vi "Database Transaction.vi"() -> ()   [LabVIEW 2013]
doc: "This VI demonstates the use of transactions on a table named transaxn in the LabVIEW.mdb database. \n\nA transaction is begun and then a table is created in the database. The user is then prompted to decide whether or not to commit the transaction and \"write\" the changes to the database."
uses:
  Auxilliary.llb/DB Tools Column Info.ctl
  Auxilliary.llb/DB Tools DataTypes.ctl
  Auxilliary.llb/DB Tools Transaction.ctl
  Connection.llb/DB Tools Open Connec (Path).vi
  Connection.llb/Conn Transaction.vi
  NI_Database_API_64.lvlib
panel:
  in  "column information":T1[](array[typedef])=[{"column name"="test", "data type"=enum."String", "size"=30, "allow null?"=FALSE}]
  in  "table":string="transaxn"
  # "INSTRUCTIONS:\n\nRun the VI.  A database connection is established and a table is created. A dialog box is then displayed asking if you want to commit or rollback the transaction."
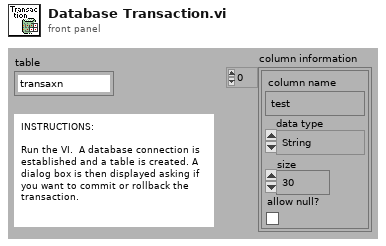
[diagram p1: front panel]
types:
  T1 = typedef "NI_Database_API_64.lvlib/DB Tools Column Info.ctl" = cluster{"column name":string, "data type":T2, "size":i32, "allow null?":bool}
  T2 = typedef "NI_Database_API_64.lvlib/DB Tools DataTypes.ctl" = enum16{"String", "Long (I32)", "Single (SGL)", "Double (DBL)", "Date/Time", "Binary"}
  T3 = typedef "NI_Database_API_64.lvlib/DB Tools Transaction.ctl" = enum16{"begin", "commit", "rollback"}
  T4 = typedef "NI_Database_API_64.lvlib/Conn ObjectReference.ctl" = refnum<k1>
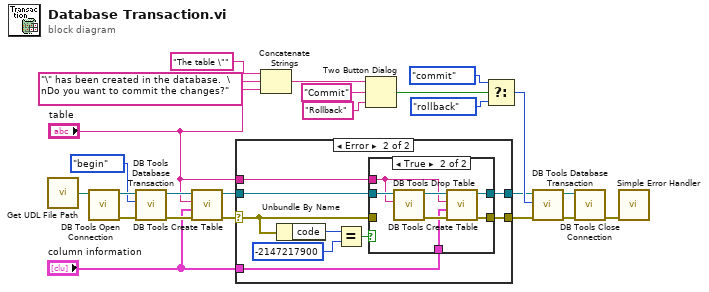
[diagram p0: block diagram]
diagram:
  n1 = call "Get UDL File Path.vi"() -> ("UDL file path"=w9:path)  [unwired: 1 in]
  n2 = call-poly "DB Tools Open Connection.vi"("connection information"=w9) -> ("error out"=w24:errorcluster, "connection reference"=w23:T4)  [unwired: 7 in]
  n3 = call-poly "DB Tools Database Transaction.vi"("error in (no error)"=w24, "operation (begin)"=DB_Tools_Transaction."begin", "connection reference"=w23) -> ("error out"=w21:errorcluster, "connection reference out"=w20:T4)  [unwired: 3 in]
  n4 = call "DB Tools Create Table.vi"("error in (no error)"=w21, "column information"="column information", "table"="table", "connection reference"=w20) -> ("error out"=w6:errorcluster, "connection reference out"=w5:T4)  [unwired: 4 in]
  n5 = case shown="Error" w6 {
    selector: w6 -> [w25 w28]
    tunnel: w5 -> [w26 w33]
    tunnel: [w26 w32] -> w4
    tunnel: [w25 w31] -> w3
    tunnel: "table" -> [_ w30]
    tunnel: "column information" -> [_ w27]
    frame No Error {
    }
    frame Error {
      n6 = Unbundle By Name(w28) -> ("code"=w35:i32)
      n7 = Equal?(x=w35, y=-2147217900) -> (x = y?=w29:bool)
      n8 = case shown="True" w29 {
        tunnel: w33 -> [w37 w44]
        tunnel: [w37 w39] -> w32
        tunnel: [w36 w38] -> w31
        tunnel: w30 -> [_ w41]
        tunnel: w28 -> [w36 _]
        tunnel: w27 -> [_ w40]
        frame False {
        }
        frame True {
          n9 = call "DB Tools Drop Table.vi"("table"=w41, "connection reference"=w44) -> ("error out"=w43:errorcluster, "connection reference out"=w42:T4)  [unwired: 6 in]
          n10 = call "DB Tools Create Table.vi"("error in (no error)"=w43, "column information"=w40, "table"=w41, "connection reference"=w42) -> ("error out"=w38:errorcluster, "connection reference out"=w39:T4)  [unwired: 4 in]
        }
      }
    }
  }
  n11 = Concatenate Strings("The table \"", "table", "\" has been created in the database.  \nDo you want to commit the changes?" ("Substring")) -> (w12:string)
  n12 = Two Button Dialog(message=w12, 1:"Rollback" ("F button name (\"Cancel\")"), 2:"Commit" ("T button name (\"OK\")")) -> (T button?=w17:bool)
  n13 = Select(t=DB_Tools_Transaction."commit" ("operation (begin)"), s=w17, f=DB_Tools_Transaction."rollback" ("operation (begin)")) -> (s? t:f=w16:T3)
  n14 = call-poly "DB Tools Database Transaction.vi"("error in (no error)"=w3, "operation (begin)"=w16, "connection reference"=w4) -> ("error out"=w19:errorcluster, "connection reference out"=w18:T4)  [unwired: 3 in]
  n15 = call "DB Tools Close Connection.vi"("error in (no error)"=w19, "connection reference"=w18) -> ("error out"=w10:errorcluster)  [unwired: 5 in]
  n16 = call <vilib>:"Simple Error Handler.vi"("error in (no error)"=w10) -> ()  [unwired: 4 in, 5 out]
